vi "Example1.vi"() -> ()   [LabVIEW 2020]
uses:
  <vilib>/Utility/miscctls.llb/LVTextColorsTypeDef.ctl
  f7be4bd8-19fd-494a-b9f8-e03963e51b59.vi
  e436cd3b-1d30-42b3-bf28-239f379a1fc4.vi
  7e30030a-63d1-4f6c-b534-7ec31a8cbec7.vi
  51baa049-ac95-47c0-b400-ff3f11f1ed40.vi
  f358dacb-5e32-4963-9fe6-18f10772d456.vi
  CtlReferences/GetAllControlRefs_Ref.vi
  CtlReferences/GetCtlValue.vi
  CtlReferences/SetCtlValue.vi
  CtlReferences/SetCtlValueSGNL.vi
  CtlReferences/GetCtlRef.vi
  CtlReferences/Error_ToSpecificClass.vi
  CtlReferences/API/Close_CtlLookup.vi
  API_Wrap/CtlReferences_API.lvlib
  CtlReferences/CtlReferences.lvclass
panel:
  in  "Colors":T1={"Text Color"=0, "Background Color"=8978407}
  in  "SetColor":bool
  out "Value":variant
  in  "GetCtl":bool
  in  "CtlName":string="Cluster.String"
  in  "NumericArray":dbl[](array[numeric])=[0.0, 1.0]
  in  "Cluster":T2={"String"="Test2", "Boolean"=FALSE, "Numeric"=12.0, "SubCluster"={"String"="Test3", "Boolean"=TRUE, "Numeric"=3.0}}
  in  "Numeric":dbl=2.0
  in  "Boolean":bool=TRUE
  in  "String":string="Test"
  in  "Stop":bool
  # "Steps:\n1. Run VI\n2. Enter valid Control Name into \"CtlName\" control\n3. Click \"Get Control Value\" to see current value displayed in \"Value\"\n4. Change colors in Colors Cluster and click Set Array Color to apply \n    to the array elements\n5. Examine Block Diagram\n\nValid Control Names:\n- Control Name\n- For Cluster elemtents : \n      ClusterName.ItemName : Cluster.String \n      ClusterName.SubCluster.ItemName : Cluster.SubCluster.String\n- For Array Elements: \n      ArrayName.Element : Array.Element"
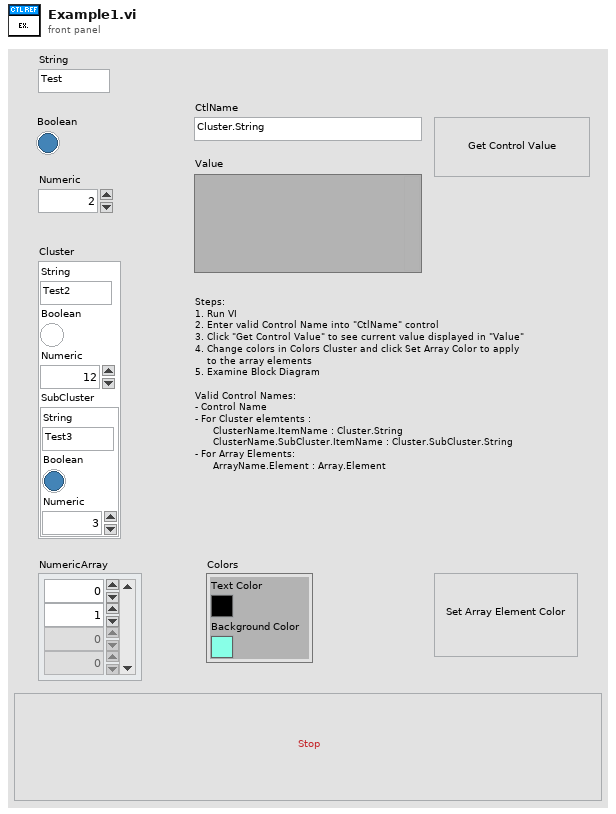
[diagram p1: front panel]
types:
  T1 = typedef "LVTextColorsTypeDef.ctl" = cluster{"Text Color":u32, "Background Color":u32}
  T2 = cluster{"String":string, "Boolean":bool, "Numeric":dbl, "SubCluster":cluster{"String":string, "Boolean":bool, "Numeric":dbl}}
  T3 = typedef "CtlReferences.lvlib/CtlReferences.lvclass/CtlLookup.ctl" = refnum<data-value>
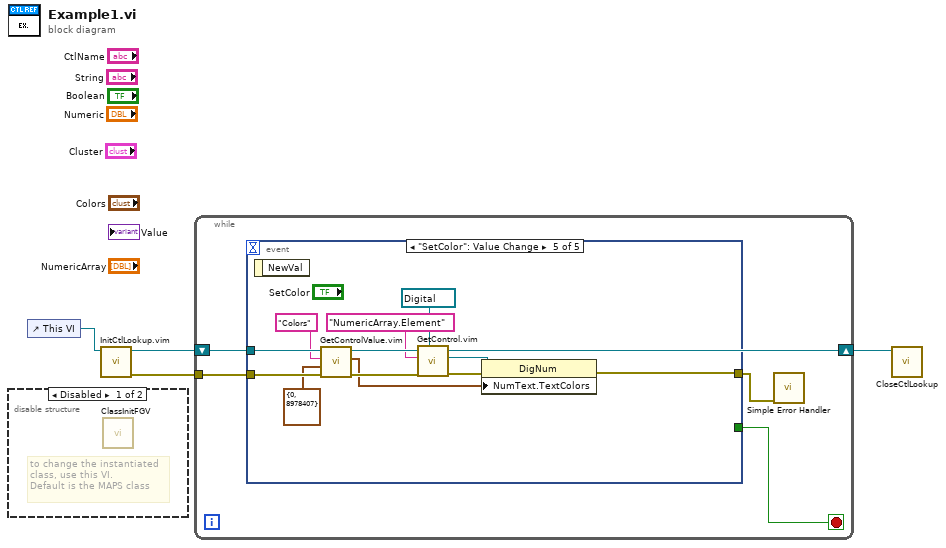
[diagram p0: block diagram]
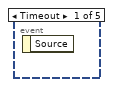
[diagram p3: hidden frame]
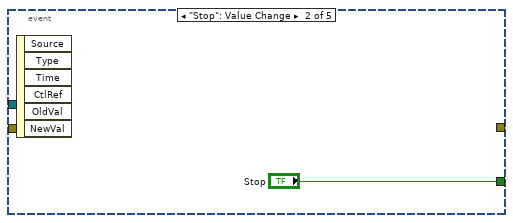
[diagram p4: hidden frame]
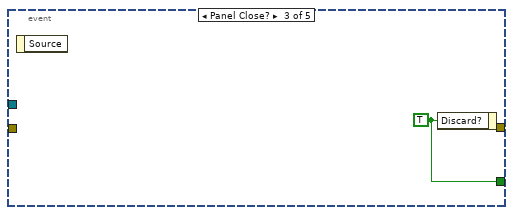
[diagram p5: hidden frame]
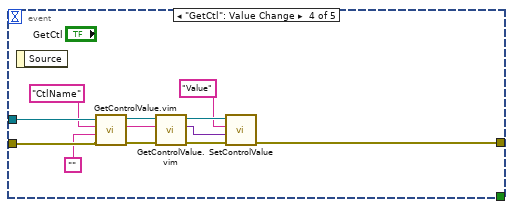
[diagram p6: hidden frame]
diagram:
  n1 = disable-structure shown="Disabled" {
    frame Disabled {
      # "to change the instantiated\nclass, use this VI.  \nDefault is the MAPS class"
      n2 = call "ClassInitFGV.vi"() -> ()  [unwired: 10 in, 2 out]
    }
    frame Enabled {
    }
  }
  n3 = control-ref of="This VI"() -> (w1:refnum<vi>)
  n4 = call "InitCtlLookup.vim"("VI Ref"=w1) -> ("error out"=w3:errorcluster, "CtlLookup Out"=w4:T3)  [unwired: 9 in]
  n5 = while {
    shift-right: [w7] -> w2
    shift-left: w4 -> [w7]
    tunnel: w3 -> [w6]
    stop <- w8 stop-if-true
    n6 = event shown="[4] \"SetColor\": Value Change" {
      selector: _ -> [_ _ _ _ _]
      dyn-events: _ -> [_ _ _ _ _]
      timeout: _ -> [_ _ _ _ _]
      tunnel: [_ "Stop" w10 _ _] -> w8
      tunnel: w7 -> [_ _ _ w22 w34]
      tunnel: w6 -> [_ _ _ w21 w33]
      tunnel: [_ _ _ w11 w23] -> w5
      event Timeout {
        n7 = event-data() -> ()  [unwired: 1 in, 1 out]
      }
      event "Stop": Value Change {
        n8 = event-data() -> ()  [unwired: 1 in, 6 out]
      }
      event Panel Close? {
        w10 = TRUE ("Discard?")
        n9 = event-data() -> ()  [unwired: 1 in, 1 out]
        n10 = event-data("Discard?"=w10) -> ()  [unwired: 1 in, 1 out]
      }
      event "GetCtl": Value Change {
        n11 = event-data() -> ()  [unwired: 1 in, 1 out]
        n12 = call "GetControlValue.vim"("error in (no error)"=w21, "Expected Data Type"="", "Control Label"="CtlName", "CtlLookup In"=w22) -> ("error out"=w18:errorcluster, "Value"=w17:string, "CtlLookup In"=w16:T3)  [unwired: 5 in]
        n13 = call "GetControlValue.vim"("error in (no error)"=w18, "Control Label"=w17, "CtlLookup In"=w16) -> ("error out"=w14:errorcluster, "Value"=w12:variant, "CtlLookup In"=w15:T3)  [unwired: 6 in]
        n14 = call "SetControlValue.vi"("error in (no error)"=w14, "Value"=w12, "Control Label"="Value", "RefCluster In"=w15) -> ("error out"=w11:errorcluster)  [unwired: 6 in, 1 out]
      }
      event "SetColor": Value Change {
        n15 = event-data() -> ()  [unwired: 1 in, 1 out]
        n16 = call "GetControlValue.vim"("error in (no error)"=w33, "Expected Data Type"=T1 {"Text Color"=0, "Background Color"=8978407} ("Colors"), "Control Label"="Colors", "CtlLookup In"=w34) -> ("error out"=w27:errorcluster, "Value"=w24:T1, "CtlLookup In"=w30:T3)  [unwired: 5 in]
        n17 = call "GetControl.vim"("Control Class"=refnum<vi> refnum, "error in (no error)"=w27, "Control Label"="NumericArray.Element", "CtlLookup In"=w30) -> ("error out"=w26:errorcluster, "Reference Out"=w25:refnum<vi>)  [unwired: 5 in, 1 out]
        n18 = property class="DigNum"(reference=w25, error in=w26, "NumText.TextColors"=w24) -> (error out=w23:errorcluster)  [unwired: 1 out]
      }
    }
    n19 = call <vilib>:"Simple Error Handler.vi"("error in (no error)"=w5) -> ()  [unwired: 4 in, 5 out]
  }
  n20 = call "CloseCtlLookup.vi"("CtlLookup In"=w2) -> ()  [unwired: 10 in, 1 out]
